vi "Excel Set Graph Font.vi"(0 "report in":refnum<class "NI_report.lvclass">, 1 "axis font":T1={"font style"="", "bold"=FALSE, "italic"=FALSE, "underline"=FALSE, "size"=0.0, "color"=4278190080} {"size" format="%.2f"}, 2 "number format (general)":string="General", 5 "axis type (xlCategory)":i32(ring)=1 items=["xlCategory"=1, "xlSeriesAxis"=3, "xlValue"=2], 9 "graph index (-1)":i16=-1, 11 "error in (no error)":errorcluster, 12 "title (\"\")":string) -> (4 "report out":refnum<class "NI_report.lvclass">, 15 "error out":errorcluster)   [LabVIEW 2010, in "NI_Excel.lvclass"]
doc: "Sets the title text and the title font of the x- and y-axes."
uses:
  <vilib>/Utility/NIReport.llb/Excel/NI_Excel.lvclass
  <vilib>/Utility/NIReport.llb/NI_report.lvclass
  <vilib>/Utility/NIReport.llb/Excel/NI_Excel.lvclass/NI_Excel.ctl
  <vilib>/addons/_office/NI_ReportGenerationToolkit.lvlib
  <vilib>/Utility/NIReport.llb/NI_ReportGenerationCore.lvlib
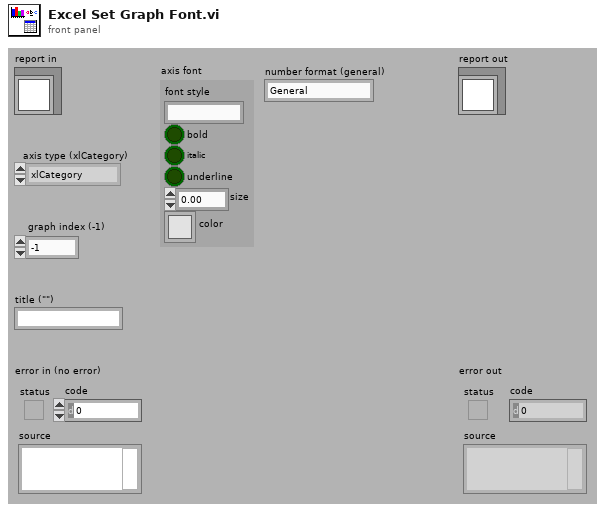
[diagram p1: front panel]
types:
  T1 = cluster{"font style":string, "bold":bool, "italic":bool, "underline":bool, "size":sgl, "color":u32}
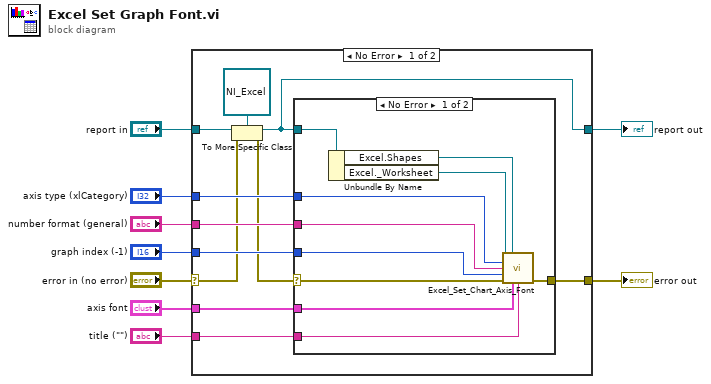
[diagram p0: block diagram]
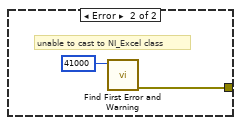
[diagram p2: hidden frame]
diagram:
  n1 = case shown="No Error" "error in (no error)" {
    selector: "error in (no error)" -> [w11 w34]
    tunnel: [w20 w34] -> w8
    tunnel: [w10 w33] -> w6
    tunnel: "report in" -> [w13 w33]
    tunnel: "axis type (xlCategory)" -> [w19 _]
    tunnel: "number format (general)" -> [w18 _]
    tunnel: "graph index (-1)" -> [w17 _]
    tunnel: "axis font" -> [w16 _]
    tunnel: "title (\"\")" -> [w15 _]
    frame No Error {
      n2 = To More Specific Class(target class=refnum<class "NI_Excel.lvclass"> refnum ("report in"), reference=w13, error in=w11) -> (specific class reference=w10:refnum<class "NI_Excel.lvclass">, error out=w12:errorcluster)
      n3 = case shown="No Error" w12 {
        selector: w12 -> [w21 _]
        tunnel: [w29 w31] -> w20
        tunnel: w19 -> [w28 _]
        tunnel: w18 -> [w27 _]
        tunnel: w17 -> [w26 _]
        tunnel: w16 -> [w25 _]
        tunnel: w15 -> [w24 _]
        tunnel: w10 -> [w22 _]
        frame No Error {
          n4 = Unbundle By Name(w22) -> ("Excel.Shapes"=w30:refnum<k7>, "Excel._Worksheet"=w23:refnum<k7>)
          n5 = call <vilib>:"Excel_Set_Chart_Axis_Font.vi"("Excel._Worksheet"=w23, "Shapes"=w30, "type"=w28, "number format"=w27, "Chart index"=w26, "error in (no error)"=w21, "axis font"=w25, "title"=w24) -> ("error out"=w29:errorcluster)  [unwired: 7 out]
        }
        frame Error {
          # "unable to cast to NI_Excel class"
          n6 = call <vilib>:"Find First Error and Warning.vi"("error code"=41000) -> ("error out"=w31:errorcluster)  [unwired: 2 in, 4 out]
        }
      }
    }
    frame Error {
    }
  }
  "error out" <- w8
  "report out" <- w6
